vi "Get Test Num.vi"(0 "Session Handle in":T1, 7 "Test Group":string, 11 "error in (no error)":errorcluster) -> (4 "Session Handle out":T1, 8 "Test Number":i32, 15 "error out":errorcluster)   [LabVIEW 2016, in "Test Number and Bin Generator.lvclass"]
uses:
  Test Number and Bin Generator.lvclass
  Typedefs/Session Handle.ctl
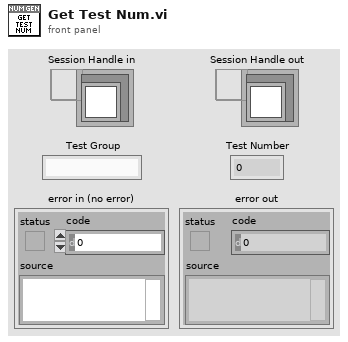
[diagram p1: front panel]
types:
  T1 = typedef "Test Number and Bin Generator.lvclass/Session Handle.ctl" = refnum<data-value>
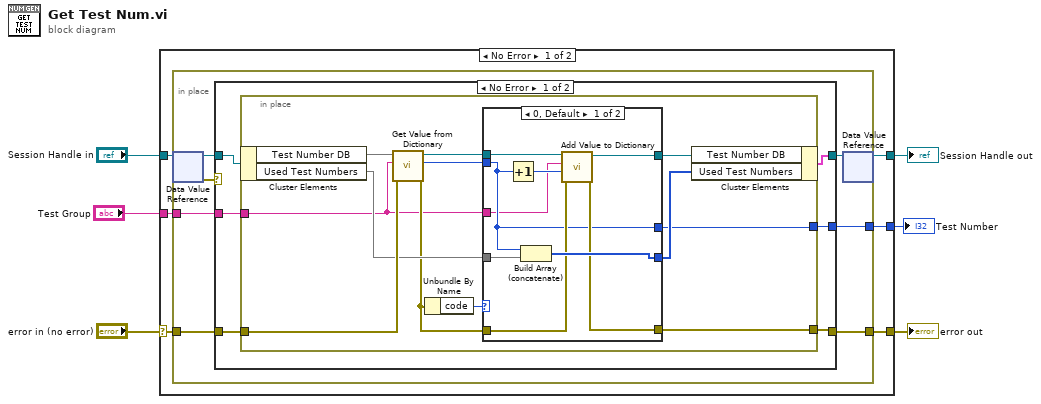
[diagram p0: block diagram]
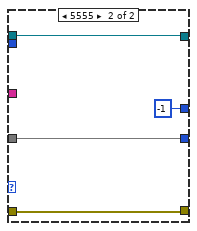
[diagram p2: hidden frame]
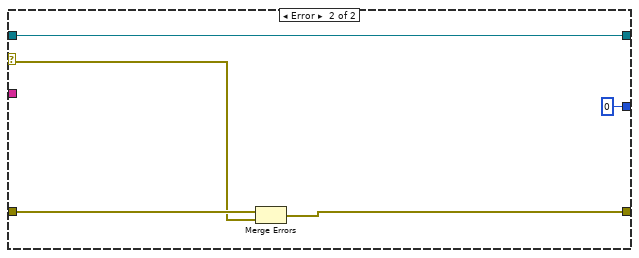
[diagram p3: hidden frame]
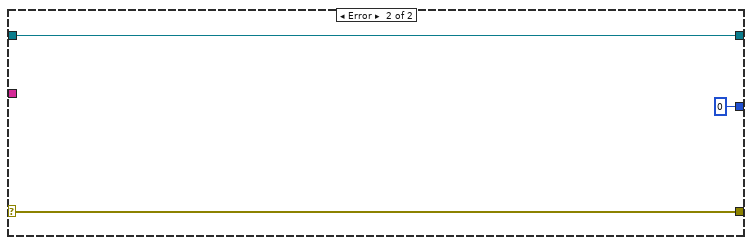
[diagram p4: hidden frame]
diagram:
  n1 = case shown="No Error" "error in (no error)" {
    selector: "error in (no error)" -> [w10 w57]
    tunnel: "Session Handle in" -> [w12 w58]
    tunnel: [w11 w58] -> w5
    tunnel: [w9 w57] -> w4
    tunnel: "Test Group" -> [w8 _]
    tunnel: [w7 0 ("Entry Value")] -> w1
    frame No Error {
      n2 = in-place {
        in-place-border: w10 -> [w15]
        in-place-border: [w18] -> w9
        in-place-border: w8 -> [w14]
        in-place-border: [w13] -> w7
        n3 = in-place-dvr #1(w12) -> (w19:refnum<class "Test Number and Bin Generator.lvclass">, w16:errorcluster)
        n4 = case shown="No Error" w16 {
          selector: w16 -> [_ w54]
          tunnel: w19 -> [w25 w52]
          tunnel: [w20 w53] -> w18
          tunnel: [w24 w52] -> w17
          tunnel: w15 -> [w23 w55]
          tunnel: w14 -> [w22 _]
          tunnel: [w21 0 ("Entry Value")] -> w13
          frame No Error {
            n5 = in-place {
              in-place-border: w23 -> [w36]
              in-place-border: w22 -> [w26]
              in-place-border: [w31] -> w21
              in-place-border: [w28] -> w20
              n6 = in-place-cluster #2(w25) -> ("Test Number DB"=w37, "Used Test Numbers"=w35)
              n7 = call "Get Value from Dictionary.vi"("error in (no error)"=w36, "Entry Name"=w26, "Integer DB In"=w37) -> ("error out"=w29:errorcluster, "Entry Value"=w32:i32, "Integer DB Out"=w33:refnum<class "Integer Dictionary.lvclass">)  [unwired: 5 in, 1 out]
              n8 = Unbundle By Name(w29) -> ("code"=w30:i32)
              n9 = case shown="0, Default" w30 {
                tunnel: w35 -> [w46 w49]
                tunnel: [w45 w49] -> w34
                tunnel: w33 -> [w44 w50]
                tunnel: w32 -> [w40 _]
                tunnel: [w40 -1 ("Entry Value")] -> w31
                tunnel: w29 -> [w43 w47]
                tunnel: [w42 w47] -> w28
                tunnel: [w41 w50] -> w27
                tunnel: w26 -> [w38 _]
                frame 0, Default {
                  n10 = Increment(x=w40) -> (x+1=w39:i32)
                  n11 = Build Array (concatenate)(w40, w46) -> (w45:i32[])
                  n12 = call "Add Value to Dictionary.vi"("error in (no error)"=w43, "Entry Value"=w39, "Entry Name"=w38, "Integer DB in"=w44) -> ("error out"=w42:errorcluster, "Integer DB out"=w41:refnum<class "Integer Dictionary.lvclass">)  [unwired: 5 in, 1 out]
                }
                frame 5555 {
                }
              }
              n13 = in-place-cluster #2("Test Number DB"=w27, "Used Test Numbers"=w34) -> (w24:cluster{})
            }
          }
          frame Error {
            n14 = Merge Errors(w55, w54) -> (w53:errorcluster)
          }
        }
        n15 = in-place-dvr #1(w17) -> (w11:T1)  [unwired: 1 out]
      }
    }
    frame Error {
    }
  }
  "Session Handle out" <- w5
  "error out" <- w4
  "Test Number" <- w1
